vi "Init.vi"(8 "error in (no error)":errorcluster, 11 "bt_Blackboard in":refnum<class "Blackboard.lvclass">) -> (0 "error out":errorcluster, 3 "bt_Blackboard out":refnum<class "Blackboard.lvclass">)   [LabVIEW 2021, in "Blackboard.lvclass"]
uses:
  Blackboard.lvclass
  Blackboard.lvclass/Blackboard.ctl
  Support/Data Type.ctl
  Support/Status Type.ctl
  Support/Data DVR Type.ctl
  Support/Tags Map Type.ctl
  Support/Group Map Type.ctl
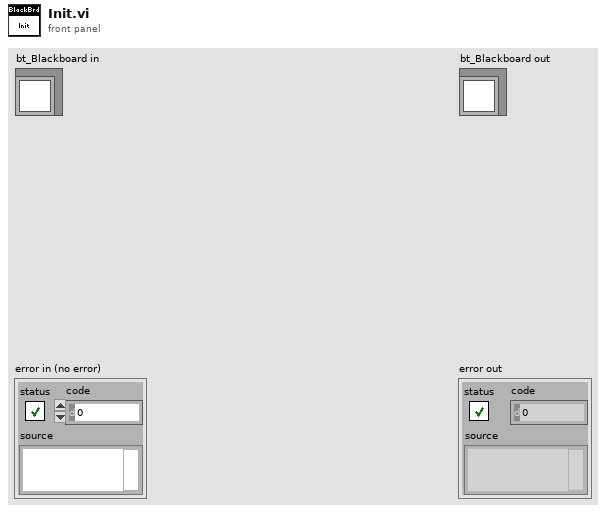
[diagram p1: front panel]
types:
  T1 = typedef "Blackboard.lvclass/Group Map Type.ctl" = map{string, i32}
  T2 = typedef "Blackboard.lvclass/Data DVR Type.ctl" = cluster{"Tags":T3, "Status":refnum<data-value>, "Boolean":refnum<data-value>, "String":refnum<data-value>, "DBL":refnum<data-value>, "SGL":refnum<data-value>, "EXT":refnum<data-value>, "U8":refnum<data-value>, "U16":refnum<data-value>, "U32":refnum<data-value>, "U64":refnum<data-value>, "I8":refnum<data-value>, "I16":refnum<data-value>, "I32":refnum<data-value>, "I64":refnum<data-value>, "CDBL":refnum<data-value>, "CSGL":refnum<data-value>, "CEXT":refnum<data-value>, "Time":refnum<data-value>, "Variant":refnum<data-value>, "Waveform":refnum<data-value>}
  T3 = typedef "Blackboard.lvclass/Tags Map Type.ctl" = map{string, cluster{"Data Index":i32, "Status Index":i32}}
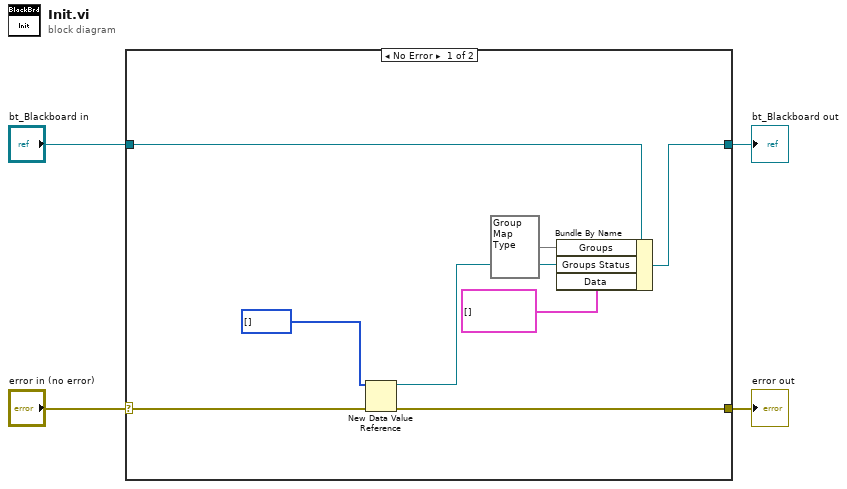
[diagram p0: block diagram]
diagram:
  n1 = case shown="No Error" "error in (no error)" {
    selector: "error in (no error)" -> [w10 w14]
    tunnel: [w7 w14] -> w3
    tunnel: [w11 w13] -> w1
    tunnel: "bt_Blackboard in" -> [w12 w13]
    frame No Error {
      n2 = New Data Value Reference(data value=i32[] [] ("Array"), error in=w10) -> (data value reference=w8:refnum<data-value>, error out=w7:errorcluster)
      n3 = Bundle By Name(cluster=w12, "Groups"=T1 {}, "Groups Status"=w8, "Data"=T2[] []) -> (w11:refnum<class "Blackboard.lvclass">)
    }
    frame Error {
    }
  }
  "error out" <- w3
  "bt_Blackboard out" <- w1
